vi "MH_SetParams.vi"(8 "error in":errorcluster, 11 "Param":T2(ring)=enum."Tous") -> (0 "error out":errorcluster)   [LabVIEW 2019]
doc: "Ce Vi enregistre les paramètres des différents axes dans un fichier .ini"
uses:
  <vilib>/Utility/config.llb/NI_LVConfig.lvlib
  <vilib>/Utility/config.llb/Write Key (Double).vi
  <vilib>/Utility/config.llb/Write Key (Boolean).vi
  <vilib>/Utility/config.llb/Write Key (String).vi
  <vilib>/Utility/config.llb/Write Key (I32).vi
  <userlib>/MultiHarp150/MH_InputChannel_LS.ctl
panel:
  in  "SyncDivider":i32(ring) caption="Divider" items=["1", "2", "4", "8", "16"]
  in  "SyncEdge":i32(ring) caption="Edge" items=["falling", "rising"]
  in  "SyncLevel":i32=-100 caption="Level (mV)" min=-1200 max=1200 step=1
  in  "SyncOffset":i32 caption="Offset (ps)" min=-100000 max=100000 step=5
  in  "UseDeadTime":bool caption="Use DT."
  in  "SyncDeadTime":i32=1000 caption="Dead T. (ps)" min=800 max=160000 step=1
  in  "Channels":T1[](array[typedef]) {"DeadTime" min=800 max=160000 step=1; "Edge" items=["falling", "rising"]; "Offset" min=-100000 max=100000 step=10; "Level" min=-1200 max=1200 step=1}
  # "Sync"
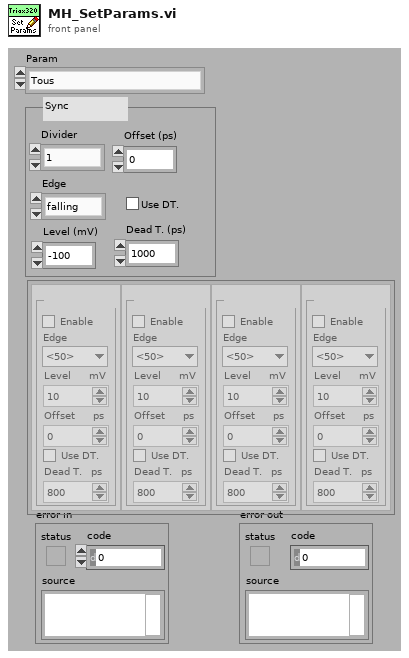
[diagram p1: front panel]
types:
  T1 = typedef "MH_InputChannel_LS.ctl" = cluster{"Name":string, "Enable":bool, "Edge":i32, "Level":i32, "Offset":i32, "UseDeadTime":bool, "DeadTime":i32}
  T2 = enum16{"Grating", "CalOffset", "Line Density (grv/mm)", "Input Slit (mm)", "Output Slit (mm)", "Both Slit (mm)", "Grating Desc.", "Wavelenght Correction", "Tous"}
  T3 = typedef "NI_LVConfig.lvlib/Config Data RefNum.ctl" = refnum<k1>
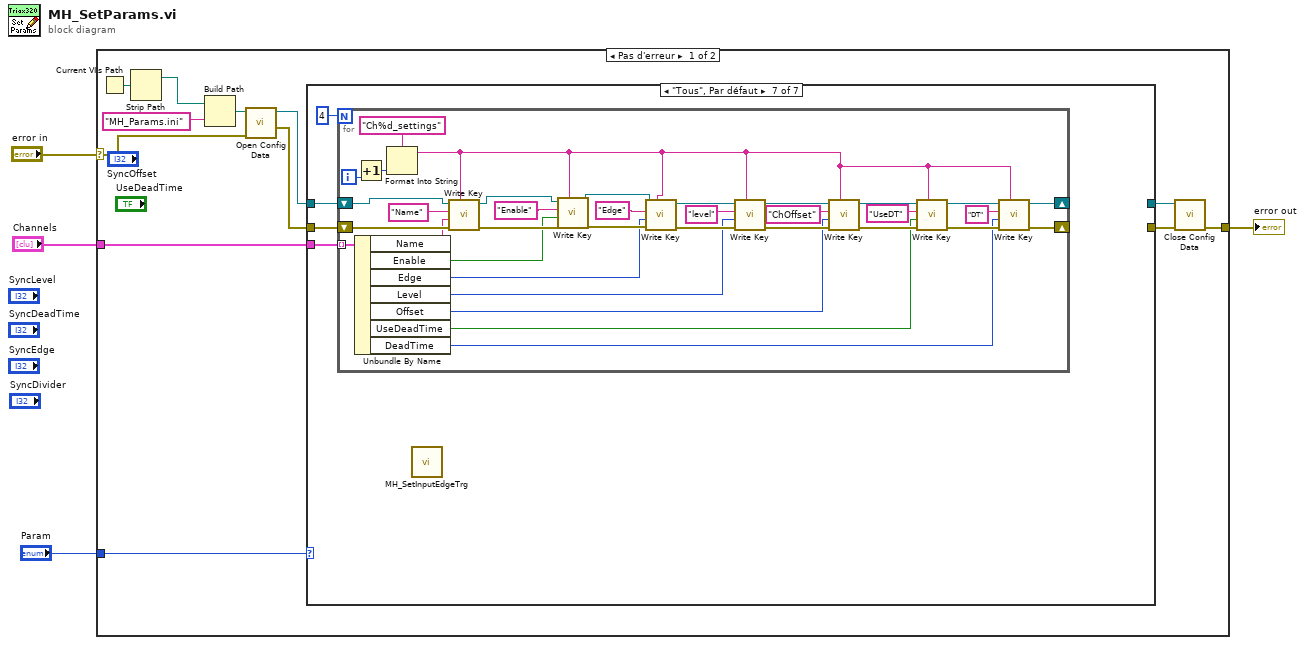
[diagram p0: block diagram]
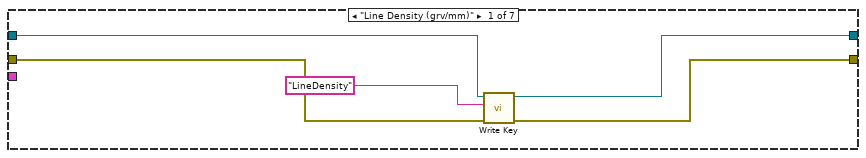
[diagram p2: hidden frame]
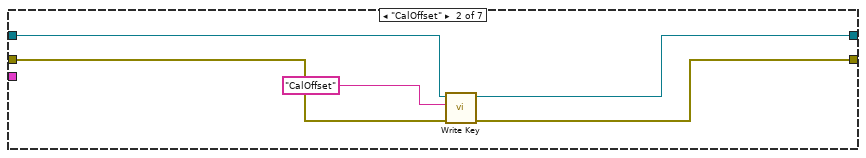
[diagram p3: hidden frame]
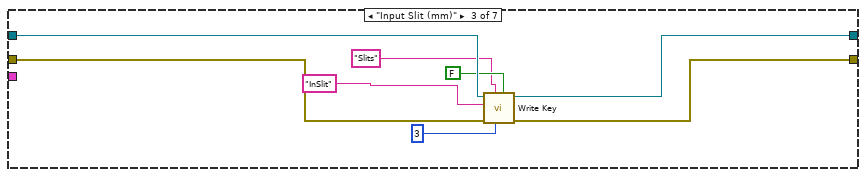
[diagram p4: hidden frame]
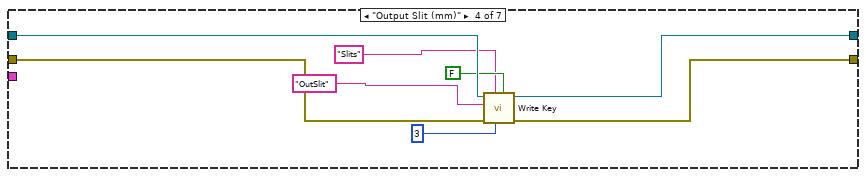
[diagram p5: hidden frame]
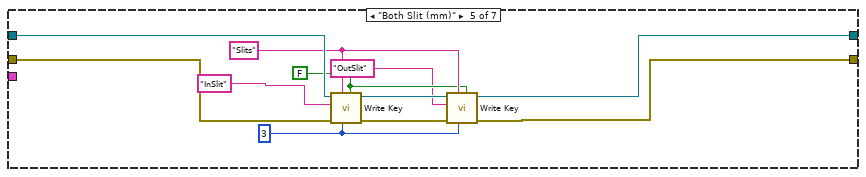
[diagram p6: hidden frame]
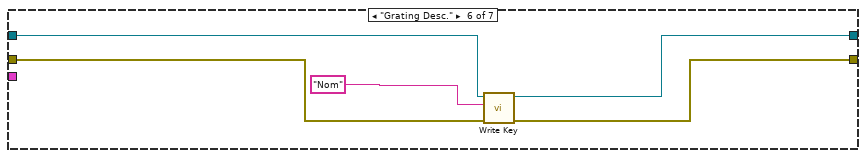
[diagram p7: hidden frame]
diagram:
  n1 = case shown="Pas d'erreur" "error in" {
    selector: "error in" -> [w6 w98]
    tunnel: [w11 w98] -> w4
    tunnel: "Param" -> [w8 _]
    tunnel: "Channels" -> [w5 _]
    frame No Error {
      n2 = Current VI's Path() -> (path=w16:path)
      n3 = Strip Path(path=w16) -> (stripped path=w7:path)  [unwired: 1 out]
      n4 = Build Path(base path=w7, name or relative path="MH_Params.ini") -> (appended path=w14:path)
      n5 = call <vilib>:"Open Config Data.vi"("error in (no error)"=w6, "configuration file path"=w14) -> ("error out"=w12:errorcluster, "refnum"=w13:T3)  [unwired: 7 in, 1 out]
      n6 = case shown="\"Tous\", Par défaut" w8 {
        tunnel: w13 -> [w19 w24 w32 w40 w53 w56 w61]
        tunnel: w12 -> [w18 w23 w31 w39 w52 w55 w62]
        tunnel: [w21 w26 w34 w42 w46 w58 _] -> w10
        tunnel: [w20 w25 w33 w41 w48 w57 _] -> w9
        tunnel: w5 -> [_ _ _ _ _ _ w59]
        frame "Line Density (grv/mm)" {
          n7 = call-poly <vilib>:"Write Key.vi"("error in (no error)"=w18, "key"="LineDensity", "refnum"=w19) -> ("error out"=w21:errorcluster, "refnum out"=w20:T3)  [unwired: 6 in, 1 out]
        }
        frame "CalOffset" {
          n8 = call-poly <vilib>:"Write Key.vi"("error in (no error)"=w23, "key"="CalOffset", "refnum"=w24) -> ("error out"=w26:errorcluster, "refnum out"=w25:T3)  [unwired: 6 in, 1 out]
        }
        frame "Input Slit (mm)" {
          n9 = call-poly <vilib>:"Write Key.vi"("use system decimal point (T)"=FALSE, "precision (6)"=i16 3, "section"="Slits", "error in (no error)"=w31, "key"="InSlit", "refnum"=w32) -> ("error out"=w34:errorcluster, "refnum out"=w33:T3)  [unwired: 3 in, 1 out]
        }
        frame "Output Slit (mm)" {
          n10 = call-poly <vilib>:"Write Key.vi"("use system decimal point (T)"=FALSE, "precision (6)"=i16 3, "section"="Slits", "error in (no error)"=w39, "key"="OutSlit", "refnum"=w40) -> ("error out"=w42:errorcluster, "refnum out"=w41:T3)  [unwired: 3 in, 1 out]
        }
        frame "Both Slit (mm)" {
          w45 = "Slits" ("section")
          w50 = i16 3 ("precision (6)")
          w44 = FALSE ("use system decimal point (T)")
          n11 = call-poly <vilib>:"Write Key.vi"("use system decimal point (T)"=w44, "precision (6)"=w50, "section"=w45, "error in (no error)"=w52, "key"="InSlit", "refnum"=w53) -> ("error out"=w49:errorcluster, "refnum out"=w47:T3)  [unwired: 3 in, 1 out]
          n12 = call-poly <vilib>:"Write Key.vi"("use system decimal point (T)"=w44, "precision (6)"=w50, "section"=w45, "error in (no error)"=w49, "key"="OutSlit", "refnum"=w47) -> ("error out"=w46:errorcluster, "refnum out"=w48:T3)  [unwired: 3 in, 1 out]
        }
        frame "Grating Desc." {
          n13 = call-poly <vilib>:"Write Key.vi"("error in (no error)"=w55, "key"="Nom", "refnum"=w56) -> ("error out"=w58:errorcluster, "refnum out"=w57:T3)  [unwired: 6 in, 1 out]
        }
        frame "Tous", Default {
          n14 = for {
            N: 4 -> [_]
            shift-right: [w89] -> _
            shift-left: w62 -> [w71]
            shift-right: [w90] -> _
            shift-left: w61 -> [w72]
            tunnel: w59 -> [w76] mode=indexing
            i -> [w79]
            n15 = Unbundle By Name(w76) -> ("Name"=w69:string, "Enable"=w68:bool, "Edge"=w67:i32, "Level"=w63:i32, "Offset"=w64:i32, "UseDeadTime"=w65:bool, "DeadTime"=w66:i32)
            n16 = Increment(x=w79) -> (x+1=w78:i32)
            n17 = Format Into String(format string="Ch%d_settings" ("section"), w78) -> (resulting string=w74:string)  [unwired: 2 in, 1 out]
            n18 = call-poly <vilib>:"Write Key.vi"("section"=w74, "error in (no error)"=w71, "value"=w69, "key"="Name", "refnum"=w72) -> ("error out"=w75:errorcluster, "refnum out"=w73:T3)  [unwired: 4 in, 1 out]
            n19 = call-poly <vilib>:"Write Key.vi"("section"=w74, "error in (no error)"=w75, "value"=w68, "key"="Enable", "refnum"=w73) -> ("error out"=w81:errorcluster, "refnum out"=w80:T3)  [unwired: 4 in, 1 out]
            n20 = call-poly <vilib>:"Write Key.vi"("section"=w74, "error in (no error)"=w81, "value"=w67, "key"="Edge", "refnum"=w80) -> ("error out"=w88:errorcluster, "refnum out"=w87:T3)  [unwired: 4 in, 1 out]
            n21 = call-poly <vilib>:"Write Key.vi"("section"=w74, "error in (no error)"=w88, "value"=w63, "key"="level", "refnum"=w87) -> ("error out"=w85:errorcluster, "refnum out"=w84:T3)  [unwired: 4 in, 1 out]
            n22 = call-poly <vilib>:"Write Key.vi"("section"=w74, "error in (no error)"=w85, "value"=w64, "key"="ChOffset", "refnum"=w84) -> ("error out"=w94:errorcluster, "refnum out"=w91:T3)  [unwired: 4 in, 1 out]
            n23 = call-poly <vilib>:"Write Key.vi"("section"=w74, "error in (no error)"=w94, "value"=w65, "key"="UseDT", "refnum"=w91) -> ("error out"=w93:errorcluster, "refnum out"=w92:T3)  [unwired: 4 in, 1 out]
            n24 = call-poly <vilib>:"Write Key.vi"("section"=w74, "error in (no error)"=w93, "value"=w66, "key"="DT", "refnum"=w92) -> ("error out"=w89:errorcluster, "refnum out"=w90:T3)  [unwired: 4 in, 1 out]
          }
          n25 = call <userlib>:"MH_SetInputEdgeTrg.vi"() -> ()  [unwired: 10 in, 2 out]
        }
      }
      n26 = call <vilib>:"Close Config Data.vi"("error in (no error)"=w10, "refnum"=w9) -> ("error out"=w11:errorcluster)  [unwired: 8 in, 1 out]
    }
    frame Error {
    }
  }
  "error out" <- w4
